vi "ReadChildren.vi"(8 "error in":errorcluster, 11 "node in":refnum<class "CEF_Node.lvclass">) -> (0 "error out":errorcluster, 2 "output array":T1[](array[typedef]), 3 "node out":refnum<class "CEF_Node.lvclass">)   [LabVIEW 2025, in "CEF.lvlib" / "CEF_Node.lvclass"]
doc: "Copyright 2017 National Instruments Corporation\n\nLicensed under the Apache License, Version 2.0 (the \"License\"); you may not use this file except in compliance with the License. You may obtain a copy of the License at http://www.apache.org/licenses/LICENSE-2.0\nUnless required by applicable law or agreed to in writing, software distributed under the License is distributed on an \"AS IS\" BASIS, WITHOUT WARRANTIES OR CONDITIONS OF ANY KIND, either express or implied. See the License for the specific language governing permissions and limitations under the License."
uses:
  CEF_Node.lvclass
  NodeRef.ctl
  CEF_Node.lvclass/CEF_Node.ctl
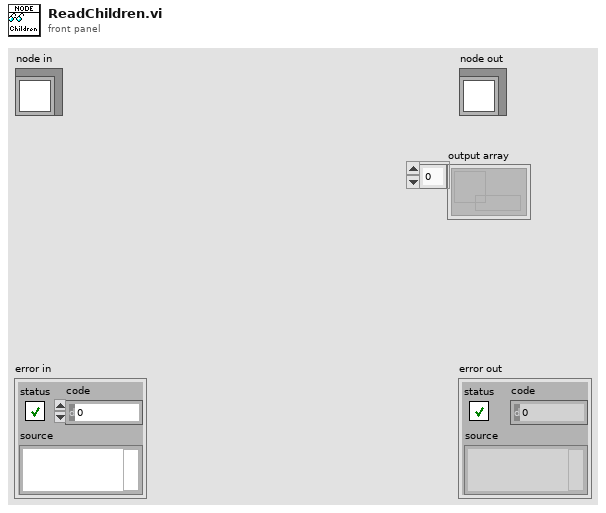
[diagram p1: front panel]
types:
  T1 = typedef "CEF.lvlib/CEF_Node.lvclass/NodeRef.ctl" = refnum<data-value>
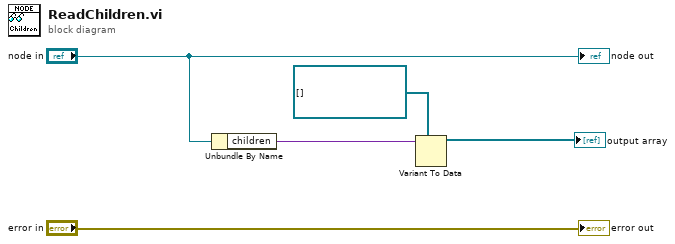
[diagram p0: block diagram]
diagram:
  n1 = Unbundle By Name("node in") -> ("children"=w3:variant)
  n2 = Variant To Data(type=refnum<data-value>[] [], Variant=w3) -> (data=→"output array":refnum<data-value>[])  [unwired: 1 in, 1 out]
  "error out" <- "error in"
  "node out" <- "node in"
